vi "Tree Control 2012 NIVerified.vi"() -> ()   [LabVIEW 2012]
doc: "This example demonstrates how to store and subsequently retrieve the hierarchy of a tree control."
panel:
  out "State":bool[](array[boolean])
  in  "randomise tree":bool
  in  "restore state":bool
  in  "save state":bool
  in  "stop":bool
  out "error out":errorcluster
  in  "error in (no error)":errorcluster
  in  "Tree":string(tree)="child 8"
  # "Overview: This example demonstrates how to store and subsequently retrieve the \nhierarchy of a tree control.\nRequirements: LabVIEW 2012 (or compatible)\nInstructions:\n1. Run the VI.\n2. Click on Randomise Tree to randomise tree structure.\n3. Click on Save State to store and display current hierarchy.\n4. Click on Restore Sated to restore the previously saved hierarchy."
  # "Save / Recall of hierarchy tree state"
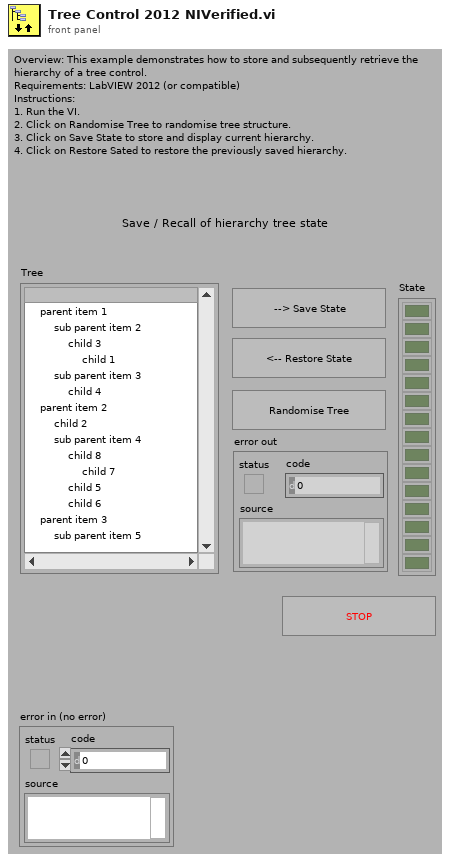
[diagram p1: front panel]
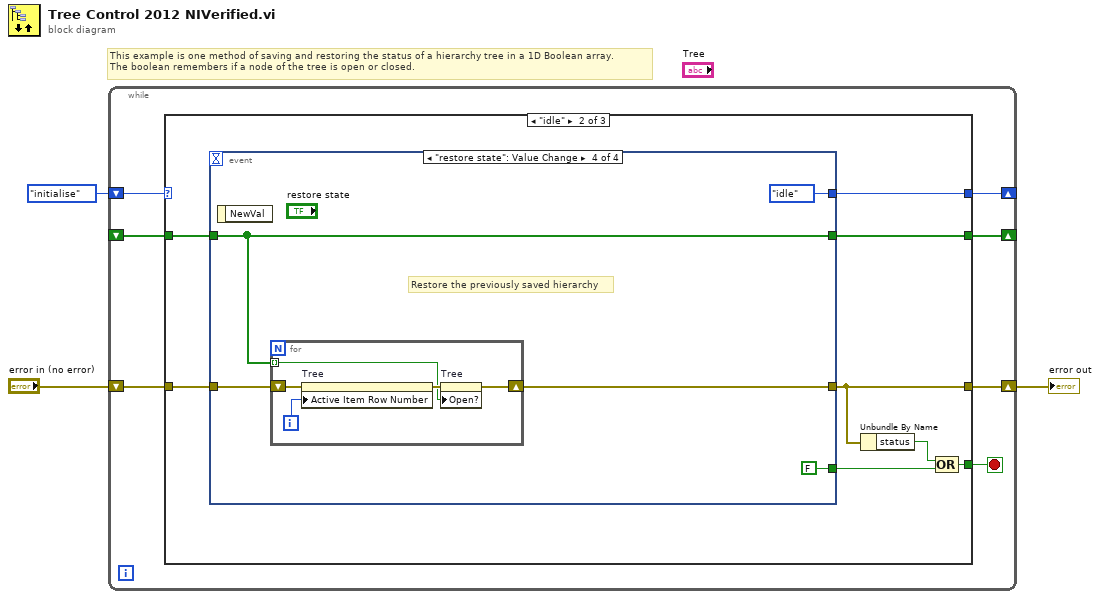
[diagram p0: block diagram]
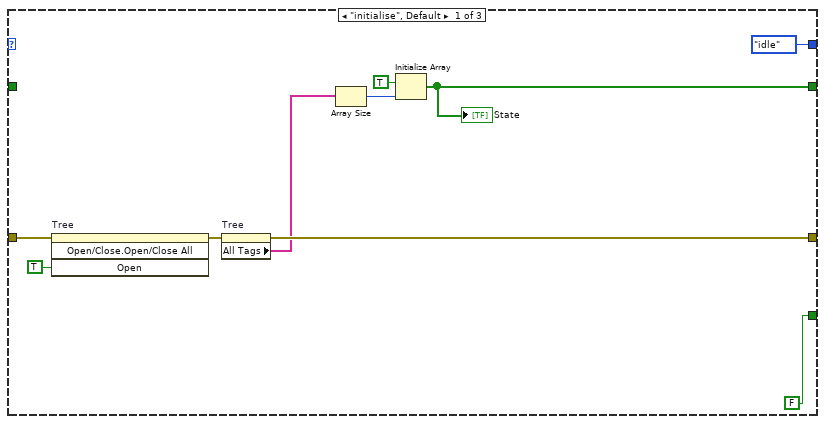
[diagram p2: hidden frame]
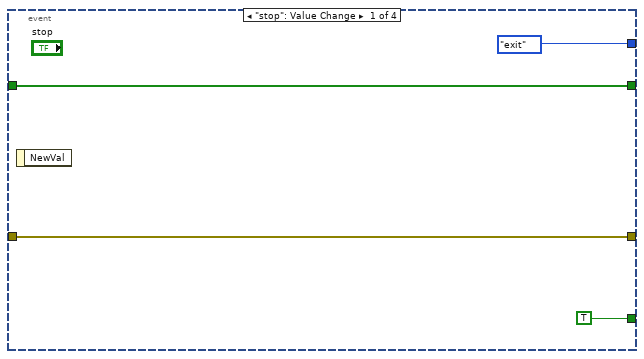
[diagram p3: hidden frame]
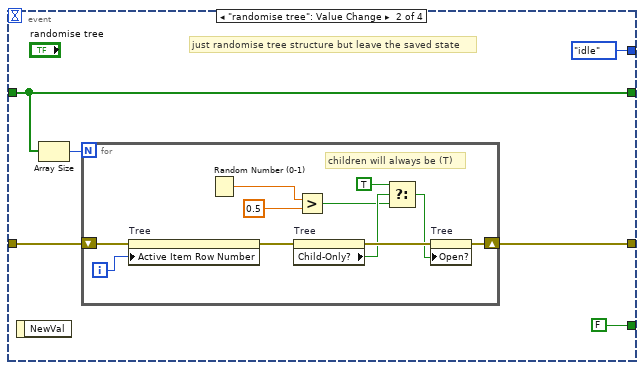
[diagram p4: hidden frame]
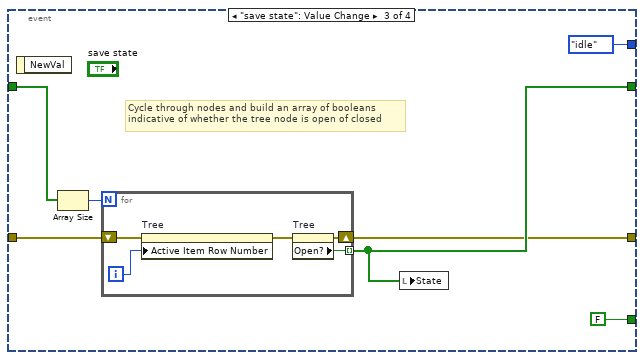
[diagram p5: hidden frame]
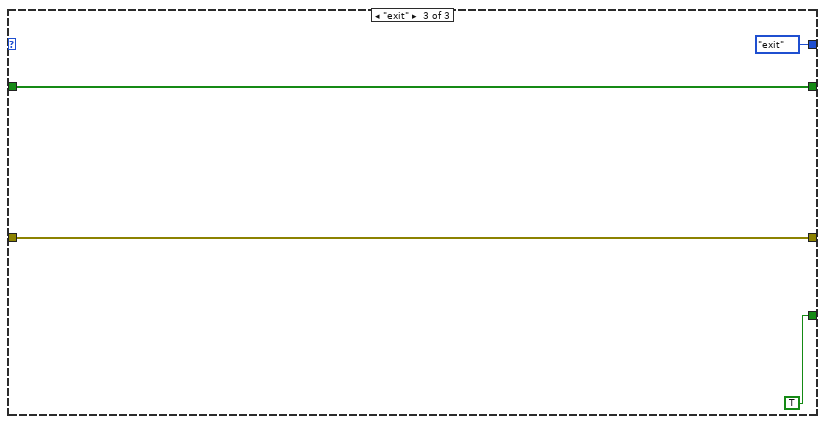
[diagram p6: hidden frame]
diagram:
  # "This example is one method of saving and restoring the status of a hierarchy tree in a 1D Boolean array.\nThe boolean remembers if a node of the tree is open or closed."
  n1 = while {
    shift-right: [w7] -> _
    shift-left: enum16{"initialise", "idle", "exit"}."initialise" -> [w10]
    shift-right: [w8] -> w1
    shift-left: "error in (no error)" -> [w9]
    shift-right: [w4] -> _
    shift-left: _ -> [w5]
    stop <- w6 stop-if-true
    n2 = case shown="\"idle\"" w10 {
      tunnel: w9 -> [w20 w27 w74]
      tunnel: [w15 w26 w74] -> w8
      tunnel: [enum16{"initialise", "idle", "exit"}."idle" w28 enum16{"initialise", "idle", "exit"}."exit"] -> w7
      tunnel: [FALSE w24 TRUE] -> w6
      tunnel: w5 -> [_ w22 w72]
      tunnel: [w11 w21 w72] -> w4
      frame "initialise", Default {
        n3 = invoke on="Tree" class="Tree (strict)" method="Open/Close.Open/Close All"(error in=w20, "Open"=TRUE ("Open?")) -> (error out=w16:errorcluster)  [unwired: 2 in, 3 out]
        n4 = property on="Tree" class="Tree (strict)"(error in=w16) -> (error out=w15:errorcluster, "All Tags"=w14:string[])  [unwired: 1 in, 1 out]
        n5 = Array Size(array=w14) -> (size(s)=w13:i32)
        n6 = Initialize Array(TRUE, w13) -> (w11:bool[])
        "State" <- w11
      }
      frame "idle" {
        n7 = event shown="[3] \"restore state\": Value Change" {
          selector: _ -> [_ _ _ _]
          dyn-events: _ -> [_ _ _ _]
          timeout: _ -> [_ _ _ _]
          tunnel: [enum16{"initialise", "idle", "exit"}."exit" enum16{"initialise", "idle", "exit"}."idle" enum16{"initialise", "idle", "exit"}."idle" enum16{"initialise", "idle", "exit"}."idle"] -> w28
          tunnel: w27 -> [w31 w35 w51 w63]
          tunnel: [w31 w34 w50 w62] -> w26
          tunnel: [TRUE FALSE FALSE FALSE] -> w23
          tunnel: w22 -> [w29 w36 w55 w64]
          tunnel: [w29 w36 w53 w64] -> w21
          event "stop": Value Change {
            n8 = event-data() -> ()  [unwired: 1 in, 1 out]
          }
          event "randomise tree": Value Change {
            # "just randomise tree structure but leave the saved state"
            n9 = event-data() -> ()  [unwired: 1 in, 1 out]
            n10 = Array Size(array=w36) -> (size(s)=w37:i32)
            n11 = for {
              N: w37 -> [_]
              shift-right: [w45] -> w34
              shift-left: w35 -> [w47]
              i -> [w46]
              # "children will always be (T)"
              n12 = property on="Tree" class="Tree (strict)"(error in=w47, "Active Item Row Number"=w46) -> (error out=w44:errorcluster)  [unwired: 1 in, 1 out]
              n13 = Random Number (0-1)() -> (number: 0 to 1=w49:dbl)
              n14 = property on="Tree" class="Tree (strict)"(error in=w44) -> (error out=w43:errorcluster, "Child-Only?"=w42:bool)  [unwired: 1 in, 1 out]
              n15 = Greater?(x=w49, y=0.5) -> (0:w41:bool)
              n16 = Select(t=TRUE, s=w42, f=w41) -> (s? t:f=w39:bool)
              n17 = property on="Tree" class="Tree (strict)"(error in=w43, "Open?"=w39) -> (error out=w45:errorcluster)  [unwired: 1 in, 1 out]
            }
          }
          event "save state": Value Change {
            # "Cycle through nodes and build an array of booleans\nindicative of whether the tree node is open of closed"
            n18 = event-data() -> ()  [unwired: 1 in, 1 out]
            n19 = Array Size(array=w55) -> (size(s)=w54:i32)
            n20 = for {
              N: w54 -> [_]
              tunnel: [w59] -> w53 mode=indexing
              shift-right: [w57] -> w50
              shift-left: w51 -> [w58]
              i -> [w61]
              n21 = property on="Tree" class="Tree (strict)"(error in=w58, "Active Item Row Number"=w61) -> (error out=w60:errorcluster)  [unwired: 1 in, 1 out]
              n22 = property on="Tree" class="Tree (strict)"(error in=w60) -> (error out=w57:errorcluster, "Open?"=w59:bool)  [unwired: 1 in, 1 out]
            }
            n23 = local write "State"(w53) -> ()
          }
          event "restore state": Value Change {
            # "Restore the previously saved hierarchy"
            n24 = event-data() -> ()  [unwired: 1 in, 1 out]
            n25 = for {
              tunnel: w64 -> [w69] mode=indexing
              shift-right: [w67] -> w62
              shift-left: w63 -> [w68]
              i -> [w71]
              n26 = property on="Tree" class="Tree (strict)"(error in=w68, "Active Item Row Number"=w71) -> (error out=w70:errorcluster)  [unwired: 1 in, 1 out]
              n27 = property on="Tree" class="Tree (strict)"(error in=w70, "Open?"=w69) -> (error out=w67:errorcluster)  [unwired: 1 in, 1 out]
            }
          }
        }
        n28 = Unbundle By Name(w26) -> ("status"=w25:bool)
        n29 = Compound Arithmetic op=OR(w25, w23) -> (w24:bool)
      }
      frame "exit" {
      }
    }
  }
  "error out" <- w1
